vi "Build Go-NoGo Pesponse.vi"(4 "error in (no error)":errorcluster, 7 "Error":T2) -> (0 "error out":errorcluster, 3 "Response":T1)   [LabVIEW 2015, in "Startup Processes.lvlib"]
uses:
  Startup Processes.lvlib
  _typedefs/Custom Remote Access Error Codes.ctl
  _typedefs/JSON Response Cluster.ctl
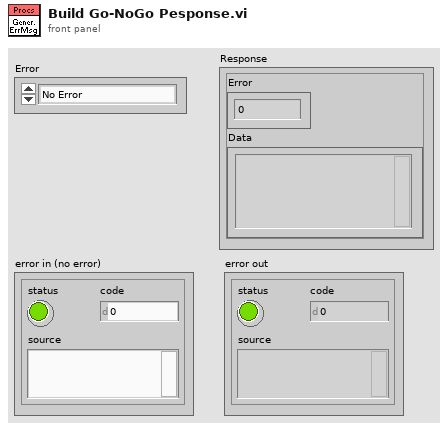
[diagram p1: front panel]
types:
  T1 = typedef "Startup Processes.lvlib/JSON Response Cluster.ctl" = cluster{"Error":i32, "Data":string}
  T2 = typedef "Startup Processes.lvlib/Custom Remote Access Error Codes.ctl" = enum16{"No Error", "CRC Error", "Update Failed"}
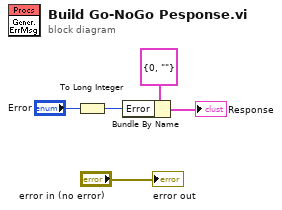
[diagram p0: block diagram]
diagram:
  n1 = To Long Integer(number="Error") -> (32bit integer=w3:i32)
  n2 = Bundle By Name(cluster=T1 {"Error"=0, "Data"=""} ("Command"), "Error"=w3) -> (→"Response":T1)
  "error out" <- "error in (no error)"
